vi "Get Payload.vi"(8 "error in (no error)":errorcluster, 11 "File Response in":refnum<class "File Response.lvclass">) -> (0 "error out":errorcluster, 2 "Payload":string, 3 "File Response out":refnum<class "File Response.lvclass">)   [LabVIEW 2020, in "HTTP Utils.lvlib" / "File Response.lvclass"]
uses:
  File Response.lvclass
  File Response.lvclass/File Response.ctl
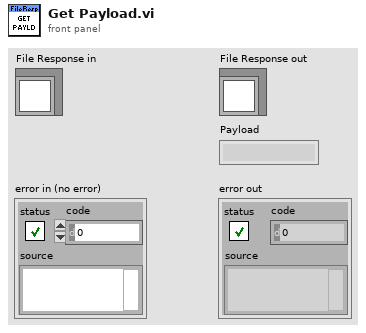
[diagram p1: front panel]
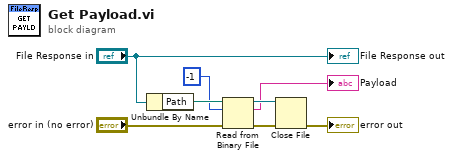
[diagram p0: block diagram]
diagram:
  n1 = Unbundle By Name("File Response in") -> ("Path"=w7:path)
  n2 = Read from Binary File(8:"error in (no error)", 10:-1 ("count (1)"), 11:w7) -> (0:w4:errorcluster, 2:→"Payload":string, 3:w5:refnum<file>)  [unwired: 3 in, 1 out]
  n3 = Close File(refnum=w5, error in=w4) -> (error out=→"error out":errorcluster)  [unwired: 1 out]
  "File Response out" <- "File Response in"
